vi "Coercion for FIRNC.vi"(6 "attenuation (db): Ar":dbl=60.0 min=0.0 format="%0.1f", 7 "ripple: rp":dbl=0.01 min=0.0 format="%0.4f", 8 "center freq: fc":dbl=0.2 min=0.0 format="%0.4f", 9 "stopband: fstop":dbl=0.02 min=0.0 format="%0.4f", 10 "passband: fpass":dbl=0.01 min=0.0 format="%0.4f", 11 "sampling freq: fs":dbl=1.0 min=0.0 format="%0.2f") -> (0 "center freq: fc":dbl format="%0.2f", 1 "stopband: fstop":dbl format="%0.2f", 2 "passband: fpass":dbl format="%0.2f", 3 "sampling freq: fs":dbl format="%0.2f", 4 "attenuation (db): Ar":dbl format="%0.2f", 5 "ripple: rp":dbl format="%0.2f")   [LabVIEW 2020, in "NI_AALBase.lvlib"]
uses:
  NI_AALBase.lvlib
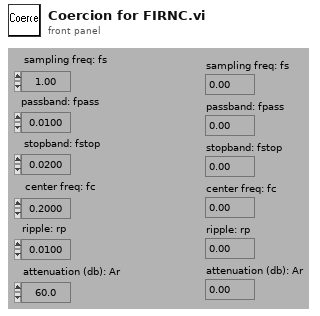
[diagram p1: front panel]
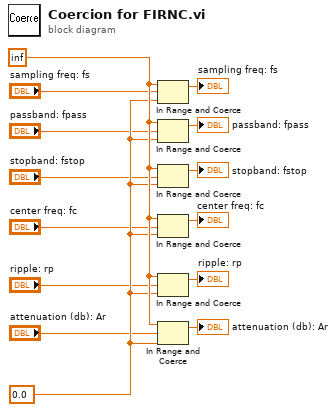
[diagram p0: block diagram]
diagram:
  w14 = inf
  w13 = 0.0
  n1 = In Range and Coerce(upper limit=w14, x="sampling freq: fs", lower limit=w13) -> (coerced(x)=→"sampling freq: fs":dbl)  [unwired: 1 out]
  n2 = In Range and Coerce(upper limit=w14, x="passband: fpass", lower limit=w13) -> (coerced(x)=→"passband: fpass":dbl)  [unwired: 1 out]
  n3 = In Range and Coerce(upper limit=w14, x="stopband: fstop", lower limit=w13) -> (coerced(x)=→"stopband: fstop":dbl)  [unwired: 1 out]
  n4 = In Range and Coerce(upper limit=w14, x="center freq: fc", lower limit=w13) -> (coerced(x)=→"center freq: fc":dbl)  [unwired: 1 out]
  n5 = In Range and Coerce(upper limit=w14, x="ripple: rp", lower limit=w13) -> (coerced(x)=→"ripple: rp":dbl)  [unwired: 1 out]
  n6 = In Range and Coerce(upper limit=w14, x="attenuation (db): Ar", lower limit=w13) -> (coerced(x)=→"attenuation (db): Ar":dbl)  [unwired: 1 out]
